vi "State.vi"(11 "Request in":refnum<class "Request.lvclass">) -> (2 "State":string)   [LabVIEW 2020, in "OAuth2.lvlib" / "Request.lvclass"]
doc: "The State string is a randomly generated code used during the OAuth2 flow to prevent spoofed requests and prevent request replay attacks on the authorization. The State code is generated and sent with the initial request and must be returned verbatim by the authorization server to confirm the redirect is in response to the intended request."
uses:
  Request.lvclass
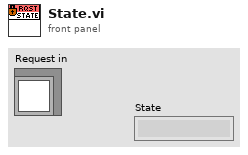
[diagram p1: front panel]
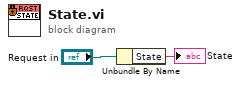
[diagram p0: block diagram]
diagram:
  n1 = Unbundle By Name("Request in") -> ("State"=→"State":string)
